vi "classification to display permissions.vi"(11 "channel classification":T1) -> (3 "permissions":T2)   [LabVIEW 2014, in "tag bus configurable plugin editor node.lvclass"]
uses:
  tag bus configurable plugin editor node.lvclass
  permissions.ctl
  <vilib>/NI/Tag Bus Module Framework/channel/channel classification.ctl
  <vilib>/NI/Tag Bus Module Framework/channel/TBM channel.lvclass
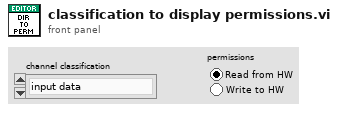
[diagram p1: front panel]
types:
  T1 = typedef "TBM channel.lvclass/channel classification.ctl" = enum16{"input data", "output data", "processing parameter", "processing result"}
  T2 = typedef "tag bus configurable plugin editor node.lvclass/permissions.ctl" = enum32{"Read from HW", "Write to HW"}
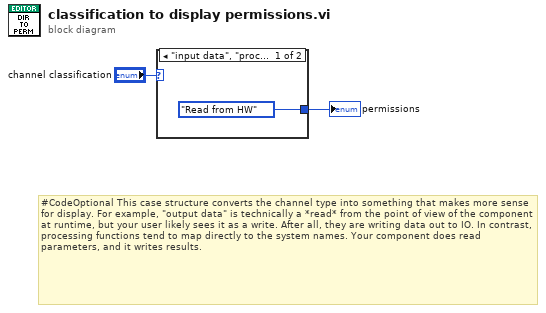
[diagram p0: block diagram]
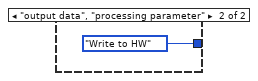
[diagram p2: hidden frame]
diagram:
  # "#CodeOptional This case structure converts the channel type into something that makes more sense for display. For example, \"output data\" is technically a *read* from the point of view of the component at runtime, but your user likely sees it as a write. After all, they are writing data out to IO. In contrast, processing functions tend to map directly to the system names. Your component does read parameters, and it writes results."
  n1 = case shown="\"input data\", \"processing result\"" "channel classification" {
    tunnel: [permissions."Read from HW" ("permissions") permissions."Write to HW" ("permissions")] -> w2
    frame "input data", "processing result" {
    }
    frame "output data", "processing parameter" {
    }
  }
  "permissions" <- w2
